vi "Process Peak Amplitude.vi"(8 "error in":errorcluster, 10 "PulseAnalysis in":T1, 11 "ChannelData in":waveform(dbl)) -> (0 "error out":errorcluster, 2 "PulseAnalysis out":T1, 3 "ChannelData Out":waveform(dbl))   [LabVIEW 2019, in "Variant Parser.lvlib" / "WaveformProcessor.lvclass"]
uses:
  Library/WaveformProcessor.lvclass
  Custom Controls/Pulse Analysis.ctl
  <vilib>/Analysis/baseanly.llb/Mean (DBL).vi
  <vilib>/measure/mascope.llb/Amplitude and Levels 1 chan.vi
  <vilib>/measure/mascope.llb/Transition Measurements 1 chan.vi
  <vilib>/Analysis/NI_AALBase.lvlib
  <vilib>/measure/NI_MAPro.lvlib
panel:
  in  "edge number (1)":i32=1 min=1
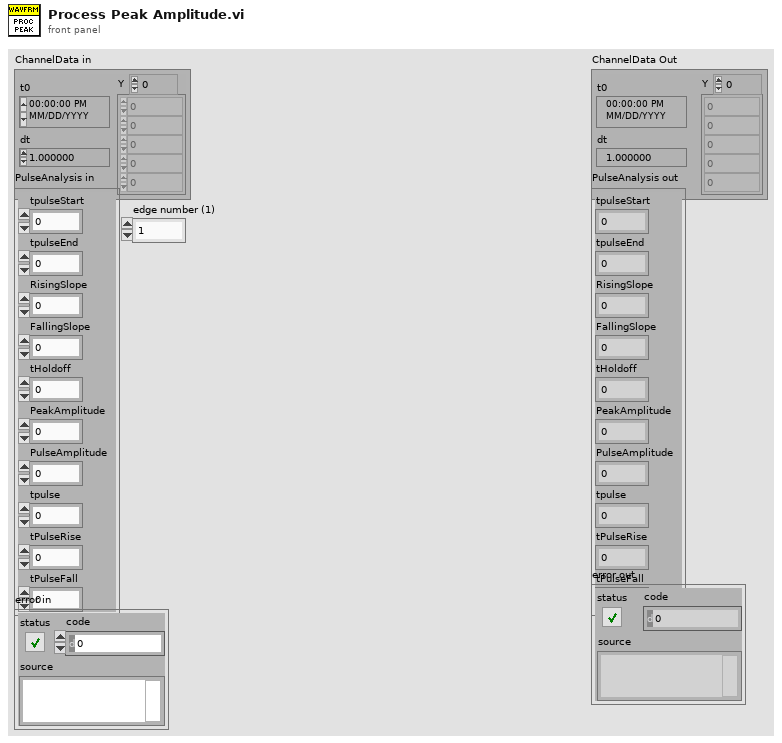
[diagram p1: front panel]
types:
  T1 = typedef "Variant Parser.lvlib/WaveformProcessor.lvclass/Pulse Analysis.ctl" = cluster{"tpulseStart":dbl, "tpulseEnd":dbl, "RisingSlope":dbl, "FallingSlope":dbl, "tHoldoff":dbl, "PeakAmplitude":dbl, "PulseAmplitude":dbl, "tpulse":dbl, "tPulseRise":dbl, "tPulseFall":dbl}
  T2 = cluster{"undershoot (%)":dbl, "overshoot (%)":dbl}
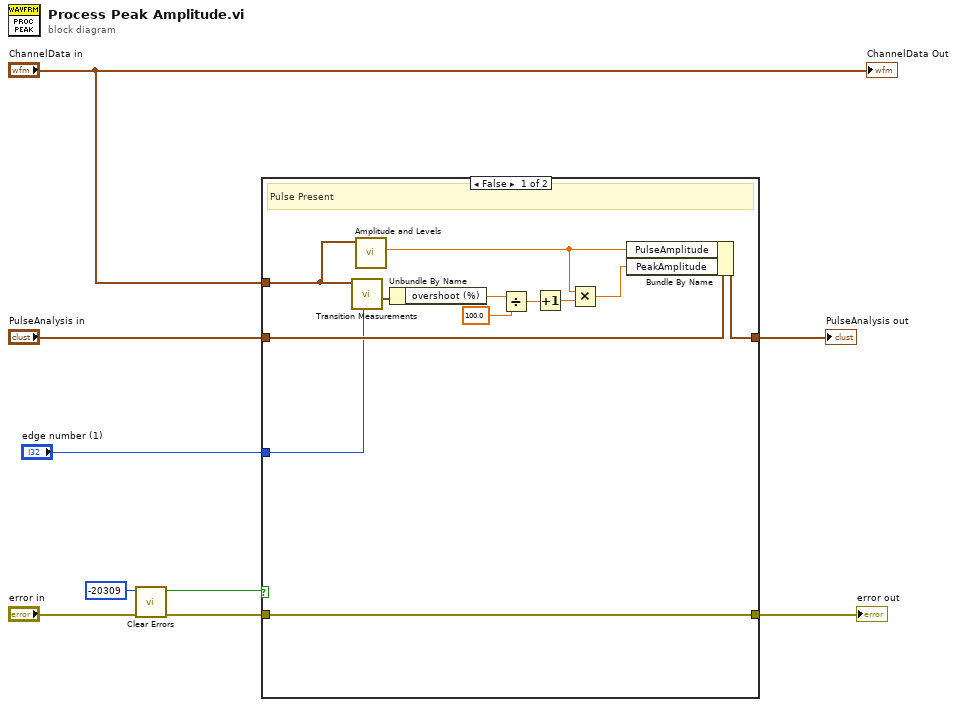
[diagram p0: block diagram]
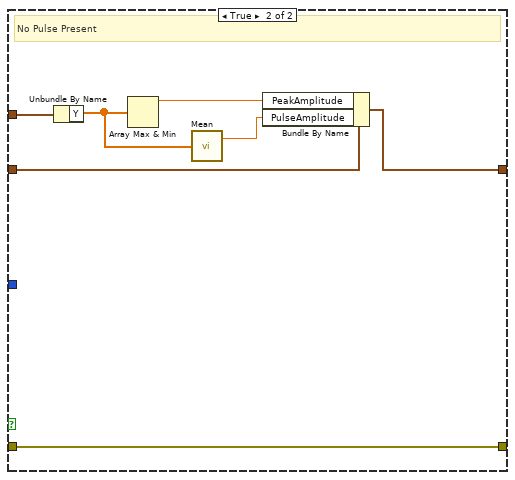
[diagram p2: hidden frame]
diagram:
  n1 = call <vilib>:"Clear Errors.vi"("error in (no error)"="error in", "specific error code to clear (0: all)"=-20309) -> ("error out"=w6:errorcluster, "specific error cleared?"=w7:bool)  [unwired: 4 in]
  n2 = case shown="False" w7 {
    tunnel: w6 -> [w20 w24]
    tunnel: "PulseAnalysis in" -> [w21 w27]
    tunnel: "ChannelData in" -> [w19 w28]
    tunnel: [w12 w26] -> w3
    tunnel: [w20 w24] -> w2
    tunnel: "edge number (1)" -> [w18 _]
    frame False {
      # "Pulse Present"
      n3 = call-poly <vilib>:"Transition Measurements.vi"("edge number (1)"=w18, "signal in"=w19) -> ("post-transition"=w17:T2)  [unwired: 4 in, 5 out]
      n4 = call-poly <vilib>:"Amplitude and Levels.vi"("signal in"=w19) -> ("high state level"=w10:dbl)  [unwired: 7 in, 3 out]
      n5 = Unbundle By Name(w17) -> ("overshoot (%)"=w16:dbl)
      n6 = Divide(x=w16, y=100.0) -> (x/y=w14:dbl)
      n7 = Increment(x=w14) -> (x+1=w13:dbl)
      n8 = Multiply(x=w10, y=w13) -> (x*y=w11:dbl)
      n9 = Bundle By Name(cluster=w21, "PulseAmplitude"=w10, "PeakAmplitude"=w11) -> (w12:T1)
    }
    frame True {
      # "No Pulse Present"
      n10 = Unbundle By Name(w28) -> ("Y"=w23:dbl[])
      n11 = Array Max & Min(array=w23) -> (max value=w25:dbl)  [unwired: 3 out]
      n12 = call-poly <vilib>:"Mean.vi"("X"=w23) -> ("mean"=w22:dbl)  [unwired: 1 out]
      n13 = Bundle By Name(cluster=w27, "PeakAmplitude"=w25, "PulseAmplitude"=w22) -> (w26:T1)
    }
  }
  "PulseAnalysis out" <- w3
  "error out" <- w2
  "ChannelData Out" <- "ChannelData in"
